vi "Send Software Start Trigger.vi"(0 "Register Bus":T1, 1 "scope":string(combo)="rx", 11 "error in":errorcluster) -> (4 "Register Bus (out)":T1, 15 "error out":errorcluster)   [LabVIEW 2017]
doc: "Send a software start trigger to the device.\n\n<B>Input Parameters</B>\n\n<B>Register Bus</B> The Register Bus object created by the ni579x Open VI and used as the session handle for the NI-579x Configuration Design Library.\n\n<B>scope</B> is the channel to send a software start trigger for. The options are \"rx\" and \"tx\".\n\n<B>error in</B> describes error conditions that occur before this node runs. This input provides standard 'error in' functionality.\n\n<B>Output Parameters</B>\n\n<B>Register Bus (out)</B> The Register Bus object created by the ni579x Open VI and used as the session handle for the NI-579x Configuration Design Library.\n\n<B>error out</B> contains error information. This output provides standard 'error out' functionality."
uses:
  <instrlib>/_niInstr/Register Bus/v0/Host/Public/Register Bus Session.ctl
  <instrlib>/_niInstr/Register Bus/v0/Host/Private/Session Data.ctl
  Rx FPGA VI Reference.ctl
  Tx FPGA VI Reference.ctl
  <vilib>/Utility/error.llb/Error Cluster From Error Code.vi
  <vilib>/rvi/errors/niLvFpgaAdjustHostInterfaceError.vi
  <vilib>/rvi/interface/nirviReadWriteControl/nirviReadWriteControl.xnode
  NiFpgaLv.dll
  <vilib>/rvi/interface/Simulation/niFpgaSimulationCallBeginRW.vi
  <instrlib>/_niInstr/Register Bus/v0/Host/niInstr Register Bus v0 Host.lvlib
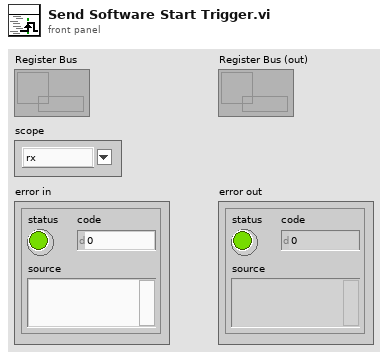
[diagram p1: front panel]
types:
  T1 = typedef "niInstr Register Bus v0 Host.lvlib/Register Bus Session.ctl" = refnum<queue>
  T2 = typedef "Rx FPGA VI Reference.ctl" = refnum<k20>
  T3 = typedef "Tx FPGA VI Reference.ctl" = refnum<k20>
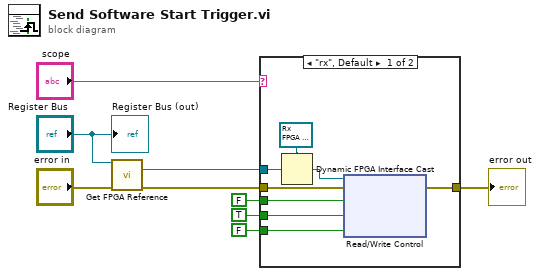
[diagram p0: block diagram]
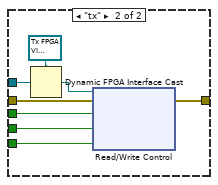
[diagram p2: hidden frame]
diagram:
  n1 = call <instrlib>:"Get FPGA Reference.vi"("session in"="Register Bus", "error in"="error in") -> ("fpga ref"=w6:refnum<k20>, "error out"=w5:errorcluster)  [unwired: 11 in, 1 out]
  n2 = case shown="\"rx\", Default" "scope" {
    tunnel: [w17 w25] -> w9
    tunnel: w6 -> [w16 w24]
    tunnel: w5 -> [w14 w22]
    tunnel: FALSE ("rf in.sw start trigger") -> [w12 w20]
    tunnel: TRUE ("rf in.sw start trigger") -> [w11 w19]
    tunnel: FALSE ("rf in.sw start trigger") -> [w10 w18]
    frame "rx", Default {
      n3 = Dynamic FPGA Interface Cast(Session In=T2 refnum ("FPGA VI Reference Out"), Type=w16) -> (Session Out=w13:T2)
      n4 = xnode "Read/Write Control"("FPGA VI Reference In"=w13, "error in"=w14, "rx.sw trigger"=w12, "rx.sw trigger"=w11, "rx.sw trigger"=w10) -> ("error out"=w17:errorcluster)  [unwired: 1 out]
    }
    frame "tx" {
      n5 = Dynamic FPGA Interface Cast(Session In=T3 refnum ("FPGA VI Reference Out"), Type=w24) -> (Session Out=w21:T3)
      n6 = xnode "Read/Write Control"("FPGA VI Reference In"=w21, "error in"=w22, "tx.sw trigger"=w20, "tx.sw trigger"=w19, "tx.sw trigger"=w18) -> ("error out"=w25:errorcluster)  [unwired: 1 out]
    }
  }
  "error out" <- w9
  "Register Bus (out)" <- "Register Bus"
